vi "Read Sensors.vi"   [LabVIEW 2019]
uses:
  Robot Global Data.vi
types:
  T1 = typedef "WPI_SwitchDevRef.ctl" = cluster{"DevStatus":errorcluster, "DIO Channel":T2, "CntIndex":T3, "Normally Closed":bool}
  T2 = typedef "FPGA_DIOChannel.ctl" = enum8{"DIO 0", "DIO 1", "DIO 2", "DIO 3", "DIO 4", "DIO 5", "DIO 6", "DIO 7", "DIO 8", "DIO 9", "DIO MXP 0", "DIO MXP 1", "DIO MXP 2", "DIO MXP 3", "DIO MXP 4", "DIO MXP 5", "DIO MXP 6", "DIO MXP 7", "DIO MXP 8", "DIO MXP 9", "DIO MXP 10", "DIO MXP 11", "DIO MXP 12", "DIO MXP 13", "DIO MXP 14", "DIO MXP 15", "SPI Port CS1", "SPI Port CS2", "SPI Port CS3", "SPI Port MISO", "SPI Port MOSI", "Invalid"}
  T3 = typedef "FPGA_CounterCtrSystemIndex.ctl" = enum8{"Ctr 0", "Ctr 1", "Ctr 2", "Ctr 3", "Ctr 4", "Ctr 5", "Ctr 6", "Ctr 7", "Invalid"}
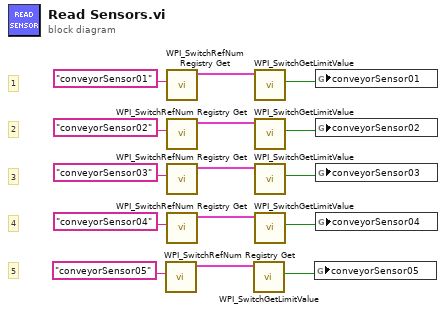
[diagram p0: block diagram]
diagram:
  # "5"
  # "4"
  # "3"
  # "2"
  # "1"
  n1 = call <vilib>:"WPI_SwitchRefNum Registry Get.vi"("refnum name"="conveyorSensor05") -> ("SwitchDevRef"=w3:T1)  [unwired: 9 in, 1 out]
  n2 = call <vilib>:"WPI_SwitchRefNum Registry Get.vi"("refnum name"="conveyorSensor01") -> ("SwitchDevRef"=w15:T1)  [unwired: 9 in, 1 out]
  n3 = call <vilib>:"WPI_SwitchRefNum Registry Get.vi"("refnum name"="conveyorSensor02") -> ("SwitchDevRef"=w12:T1)  [unwired: 9 in, 1 out]
  n4 = call <vilib>:"WPI_SwitchRefNum Registry Get.vi"("refnum name"="conveyorSensor03") -> ("SwitchDevRef"=w9:T1)  [unwired: 9 in, 1 out]
  n5 = call <vilib>:"WPI_SwitchRefNum Registry Get.vi"("refnum name"="conveyorSensor04") -> ("SwitchDevRef"=w6:T1)  [unwired: 9 in, 1 out]
  n6 = call <vilib>:"WPI_SwitchGetLimitValue.vi"("SwitchDevRef"=w3) -> ("Switch Pressed"=w1:bool)  [unwired: 8 in, 2 out]
  n7 = call <vilib>:"WPI_SwitchGetLimitValue.vi"("SwitchDevRef"=w15) -> ("Switch Pressed"=w13:bool)  [unwired: 8 in, 2 out]
  n8 = call <vilib>:"WPI_SwitchGetLimitValue.vi"("SwitchDevRef"=w12) -> ("Switch Pressed"=w10:bool)  [unwired: 8 in, 2 out]
  n9 = call <vilib>:"WPI_SwitchGetLimitValue.vi"("SwitchDevRef"=w9) -> ("Switch Pressed"=w7:bool)  [unwired: 8 in, 2 out]
  n10 = call <vilib>:"WPI_SwitchGetLimitValue.vi"("SwitchDevRef"=w6) -> ("Switch Pressed"=w4:bool)  [unwired: 8 in, 2 out]
  n11 = global write "Robot Global Data.vi" "conveyorSensor05"(w1) -> ()
  n12 = global write "Robot Global Data.vi" "conveyorSensor01"(w13) -> ()
  n13 = global write "Robot Global Data.vi" "conveyorSensor02"(w10) -> ()
  n14 = global write "Robot Global Data.vi" "conveyorSensor03"(w7) -> ()
  n15 = global write "Robot Global Data.vi" "conveyorSensor04"(w4) -> ()
